vi "Get All Status Interface Info.vi"(8 "error in (no error)":errorcluster, 11 "CSM-Helper in":refnum<class "CSM-Helper.lvclass">) -> (0 "error out":errorcluster, 2 "Array 3":cluster{string, "Argument":T1}[](array[cluster]), 3 "CSM-Helper out":refnum<class "CSM-Helper.lvclass">)   [LabVIEW 2017, in "CSM-Helper.lvclass"]
doc: "### Get All Status Interface Info.vi\n\n-- <b>Controls</b> --\n- <b>CSM-Helper in</b>: CSMHelper input\n\n-- <b>Indicators</b> --\n- <b>Array 3</b>:\n- <b>CSM-Helper out</b>: CSMHelper output"
uses:
  CSM-Helper.lvclass
  Typedef/Def-Argument Info.ctl
  CSM-Helper.lvclass/CSM-Helper.ctl
  <vilib>/Utility/traverseref.llb/TRef TravTarget.ctl
  <vilib>/Utility/traverseref.llb/VI Scripting - Traverse.lvlib
  Utility/_Support/Terminals.llb/csmHelper-Terminals.lvlib
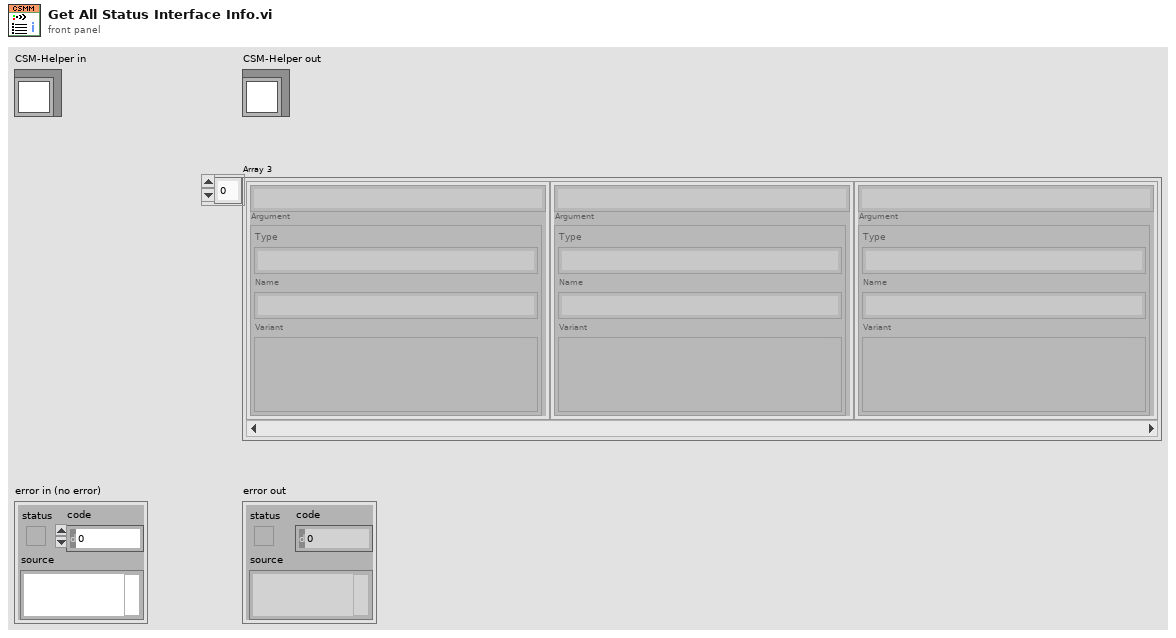
[diagram p1: front panel]
types:
  T1 = typedef "CSM-Helper.lvclass/Def-Argument Info.ctl" = cluster{"Type":string, "Name":string, "Variant":variant}
  T2 = typedef "TRef TravTarget.ctl" = enum16{"FP", "BD", "Other"}
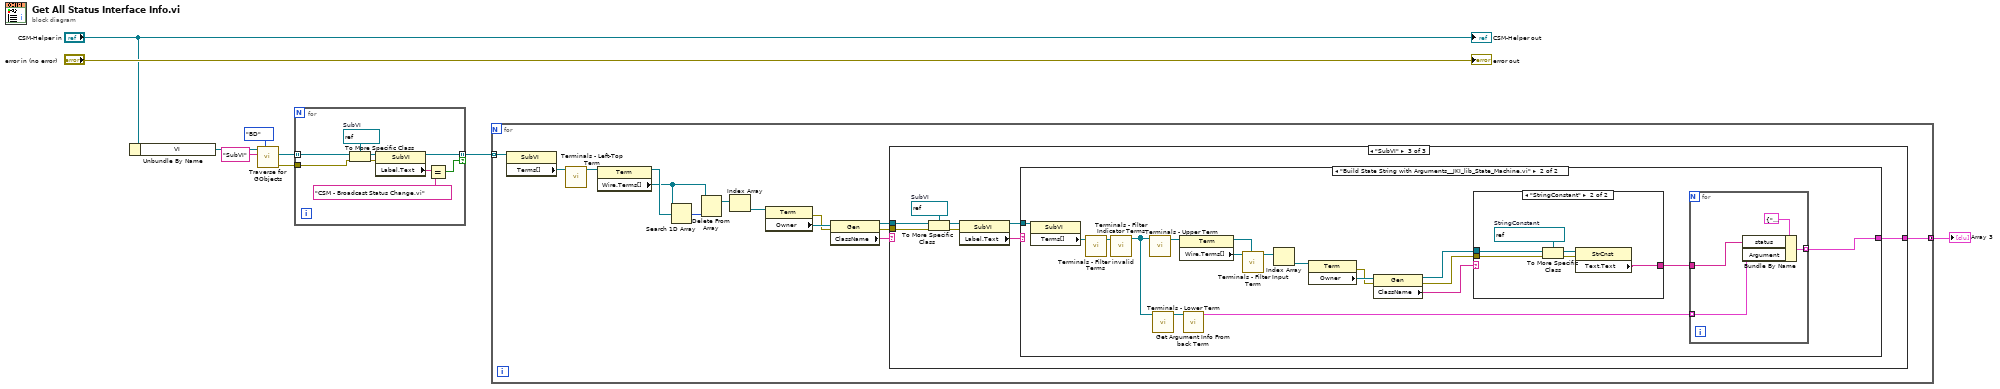
[diagram p0: block diagram]
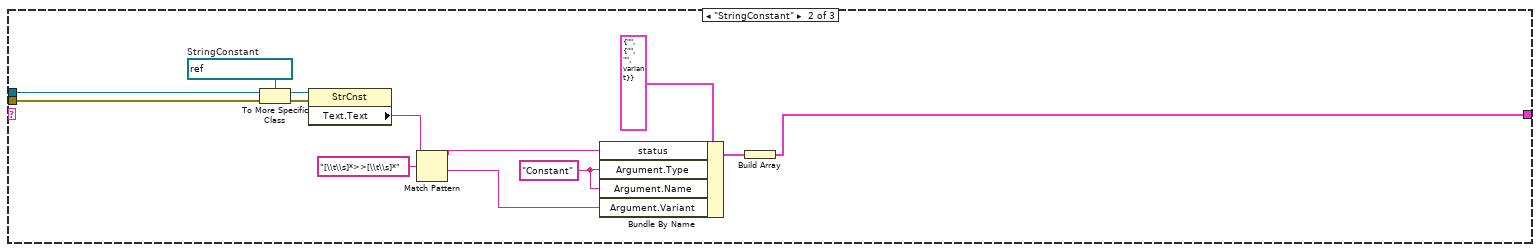
[diagram p3: hidden frame]
diagram:
  n1 = Unbundle By Name("CSM-Helper in") -> ("VI"=w2:refnum<vi>)
  n2 = call <vilib>:"Traverse for GObjects.vi"("Traverse Target"=TRef_TravTarget."BD", "Class Name"="SubVI", "VI Refnum"=w2) -> ("error out"=w4:errorcluster, "References"=w5:refnum<vi>[])  [unwired: 5 in, 2 out]
  n3 = for {
    tunnel: w5 -> [w18] mode=indexing
    tunnel: w4 -> [w14]
    tunnel: [w11] -> w3 mode=indexing if=w10
    w15 = refnum<vi> refnum  # SubVI
    n4 = To More Specific Class(target class=w15, reference=w18, error in=w14) -> (specific class reference=w17:refnum<vi>, error out=w16:errorcluster)
    n5 = property class="SubVI"(reference=w17, error in=w16) -> (reference out=w11:refnum<vi>, "Label.Text"=w13:string)  [unwired: 1 out]
    n6 = Equal?(x=w13, y="CSM - Broadcast Status Change.vi") -> (x = y?=w10:bool)
  }
  n7 = for {
    tunnel: w3 -> [w32] mode=indexing
    tunnel: [w19] -> w1 mode=concatenating
    n8 = property class="SubVI"(reference=w32) -> ("Terms[]"=w31:refnum<vi>[])  [unwired: 1 in, 2 out]
    n9 = call "Terminals - Left-Top Term.vi"("Terms[]"=w31) -> ("Terms[] out"=w30:refnum<vi>)  [unwired: 10 in]
    n10 = property class="Term"(reference=w30) -> (reference out=w29:refnum<vi>, "Wire.Terms[]"=w27:refnum<vi>[])  [unwired: 1 in, 1 out]
    n11 = Search 1D Array(1D array=w27, element=w29) -> (index of element=w28:i32)  [unwired: 1 in]
    n12 = Delete From Array(array=w27, index=w28) -> (array with subset deleted=w26:refnum<vi>[])  [unwired: 1 in, 1 out]
    n13 = Index Array(array=w26) -> (element=w25:refnum<vi>)  [unwired: 1 in]
    n14 = property class="Term"(reference=w25) -> (error out=w23:errorcluster, "Owner"=w24:refnum<vi>)  [unwired: 1 in, 1 out]
    n15 = property class="Gen"(reference=w24, error in=w23) -> (reference out=w21:refnum<vi>, error out=w20:errorcluster, "ClassName"=w22:string)
    n16 = case shown="\"SubVI\"" w22 {
      tunnel: w21 -> [_ w45 w53]
      tunnel: w20 -> [_ w43 w51]
      tunnel: [_ w33 w46] -> w19
      frame "False", Default {
      }
      frame "StringConstant" {
        w35 = "Constant" ("Argument.Type")
        w41 = refnum<vi> refnum  # StringConstant
        n17 = To More Specific Class(target class=w41, reference=w45, error in=w43) -> (specific class reference=w44:refnum<vi>, error out=w42:errorcluster)
        n18 = property class="StrCnst"(reference=w44, error in=w42) -> ("Text.Text"=w40:string)  [unwired: 2 out]
        n19 = Match Pattern(string=w40, regular expression="[\\t\\s]*>>[\\t\\s]*") -> (before substring=w36:string, after substring=w34:string)  [unwired: 1 in, 2 out]
        n20 = Bundle By Name(cluster=cluster{"status":string, "Argument":T1} {"status"="", "Argument"={"Type"="", "Name"="", "Variant"=variant}}, "status"=w36, "Argument.Type"=w35, "Argument.Name"=w35, "Argument.Variant"=w34) -> (w37:cluster{"status":string, "Argument":T1})
        n21 = Build Array(w37) -> (w33:cluster{"status":string, "Argument":T1}[])
      }
      frame "SubVI" {
        w49 = refnum<vi> refnum  # SubVI
        n22 = To More Specific Class(target class=w49, reference=w53, error in=w51) -> (specific class reference=w52:refnum<vi>, error out=w50:errorcluster)
        n23 = property class="SubVI"(reference=w52, error in=w50) -> (reference out=w47:refnum<vi>, "Label.Text"=w48:string)  [unwired: 1 out]
        n24 = case shown="\"Build State String with Arguments__JKI_lib_State_Machine.vi\"" w48 {
          tunnel: w47 -> [_ w71]
          tunnel: [_ w60] -> w46
          frame Default {
          }
          frame "Build State String with Arguments__JKI_lib_State_Machine.vi" {
            n25 = property class="SubVI"(reference=w71) -> ("Terms[]"=w70:refnum<vi>[])  [unwired: 1 in, 2 out]
            n26 = call "Terminals - Filter invalid Terms.vi"("Terms[]"=w70) -> ("Terms[] out"=w62:refnum<vi>[])  [unwired: 10 in]
            n27 = call "Terminals - Filter Indicator Terms.vi"("Terms[]"=w62) -> ("Terms[] out"=w56:refnum<vi>[])  [unwired: 10 in]
            n28 = call "Terminals - Upper Term.vi"("Terms[]"=w56) -> ("Terms[] out"=w66:refnum<vi>)  [unwired: 10 in]
            n29 = call "Terminals - Lower Term.vi"("Terms[]"=w56) -> ("Terms[] out"=w54:refnum<vi>)  [unwired: 10 in]
            n30 = property class="Term"(reference=w66) -> (reference out=w58:refnum<vi>, "Wire.Terms[]"=w59:refnum<vi>[])  [unwired: 1 in, 1 out]
            n31 = call "Get Argument Info From back Term.vi"("Terminal in"=w54) -> ("Array"=w55:T1[])  [unwired: 10 in]
            n32 = call "Terminals - Filter Input Term.vi"("InnerTerminal in"=w58, "Wire.Terms[] in"=w59) -> ("Wire.Terms[] out"=w57:refnum<vi>[])  [unwired: 9 in]
            n33 = Index Array(array=w57) -> (element=w69:refnum<vi>)  [unwired: 1 in]
            n34 = property class="Term"(reference=w69) -> (error out=w67:errorcluster, "Owner"=w68:refnum<vi>)  [unwired: 1 in, 1 out]
            n35 = property class="Gen"(reference=w68, error in=w67) -> (reference out=w63:refnum<vi>, error out=w64:errorcluster, "ClassName"=w65:string)
            n36 = case shown="\"StringConstant\"" w65 {
              tunnel: w63 -> [_ w81]
              tunnel: w64 -> [_ w79]
              tunnel: [_ w76] -> w61
              frame Default {
              }
              frame "StringConstant" {
                w77 = refnum<vi> refnum  # StringConstant
                n37 = To More Specific Class(target class=w77, reference=w81, error in=w79) -> (specific class reference=w80:refnum<vi>, error out=w78:errorcluster)
                n38 = property class="StrCnst"(reference=w80, error in=w78) -> ("Text.Text"=w76:string)  [unwired: 2 out]
              }
            }
            n39 = for {
              tunnel: w61 -> [w74]
              tunnel: [w73] -> w60 mode=indexing
              tunnel: w55 -> [w72] mode=indexing
              n40 = Bundle By Name(cluster=cluster{"status":string, "Argument":T1} {"status"="", "Argument"={"Type"="", "Name"="", "Variant"=variant}}, "status"=w74, "Argument"=w72) -> (w73:cluster{"status":string, "Argument":T1})
            }
          }
        }
      }
    }
  }
  "Array 3" <- w1
  "error out" <- "error in (no error)"
  "CSM-Helper out" <- "CSM-Helper in"
